vi "Pass State Machine.vi"   [LabVIEW 2013]
uses:
  typedefs/fg_typedef.ctl
  typedefs/subStates.ctl
  typedefs/DevRef Type.ctl
panel:
  # "A State Machine to Handle Passing"
types:
  T1 = typedef "subStates.ctl" = enum16{"null", "wait", "driver control", "auto", "manual override", "hold position", "rotate", "pickup", "pass", "load", "goto shoot", "shoot high goal", "shoot low goal", "cancel arm", "cancel shooter", "end"}
  T2 = typedef "fg_typedef.ctl" = enum16{"Get", "Set"}
  T3 = typedef "DevRef Type.ctl" = enum16{"Shooter Solenoid", "Latch Solenoid", "Right Up Sensor", "Right Down Sensor", "Hold Sensor", "2 Ball Switch", "Arm Encoder"}
  T4 = typedef "WPI_DigitalInputDevRef.ctl" = cluster{"DevStatus":errorcluster, "DIO Channel":T5, "Digital Module":T6}
  T5 = typedef "FPGA_DIOChannel.ctl" = enum8{"DIO 1", "DIO 2", "DIO 3", "DIO 4", "DIO 5", "DIO 6", "DIO 7", "DIO 8", "DIO 9", "DIO 10", "DIO 11", "DIO 12", "DIO 13", "DIO 14", "Invalid"}
  T6 = typedef "FPGA_TypedefDigitalModule.ctl" = enum16{"Digital Module 1", "Digital Module 2"}
  T7 = typedef "WPI_EncoderDevRef.ctl" = cluster{"DevStatus":errorcluster, "EncoderIndex":T8, "CounterIndex":T9, "DistancePerCount":dbl, "Decoding Type":T10}
  T8 = typedef "FPGA_EncoderIdx.ctl" = enum8{"Enc 0", "Enc 1", "Enc 2", "Enc 3", "Invalid"}
  T9 = typedef "FPGA_CounterCtrSystemIndex.ctl" = enum8{"Ctr 0", "Ctr 1", "Ctr 2", "Ctr 3", "Ctr 4", "Ctr 5", "Ctr 6", "Ctr 7", "Invalid"}
  T10 = typedef "WPI_EncoderType.ctl" = enum16{"1x", "2x", "4x"}
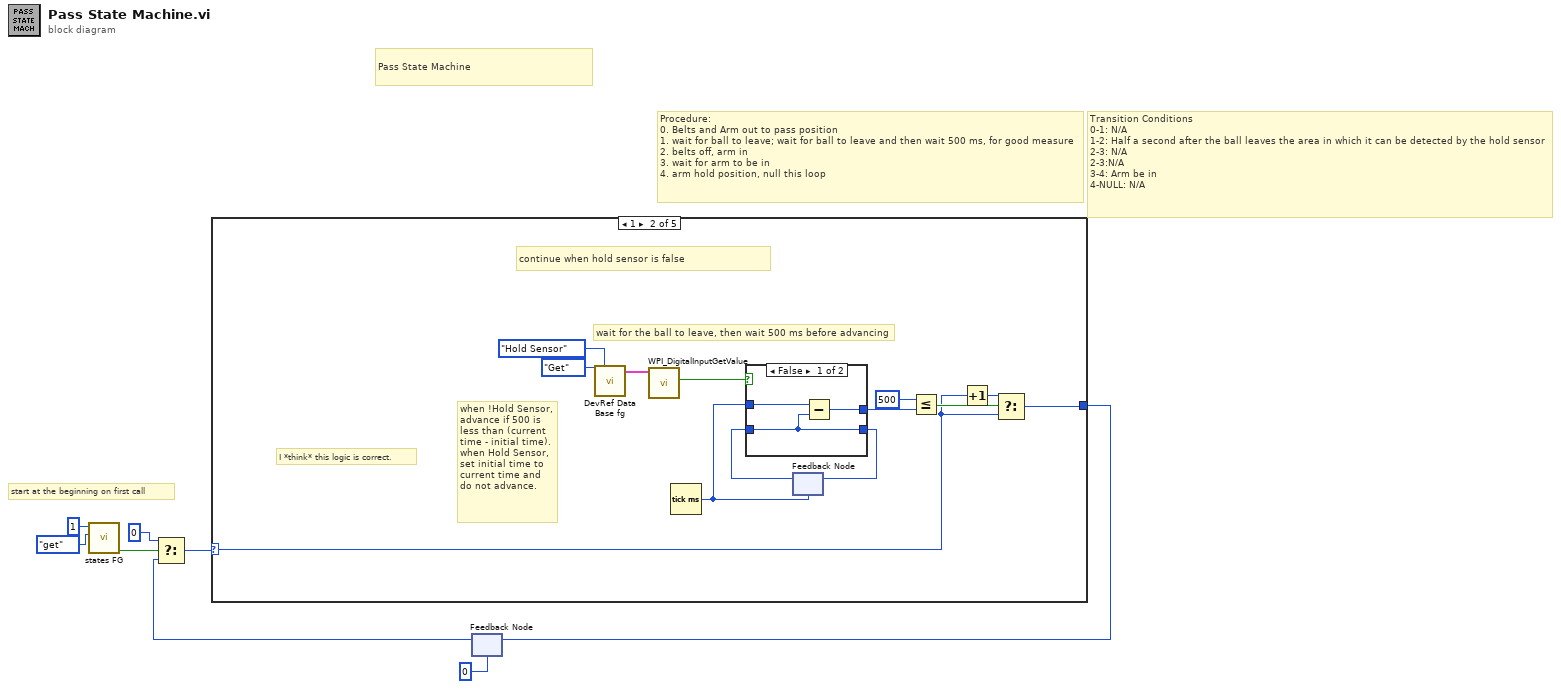
[diagram p0: block diagram]
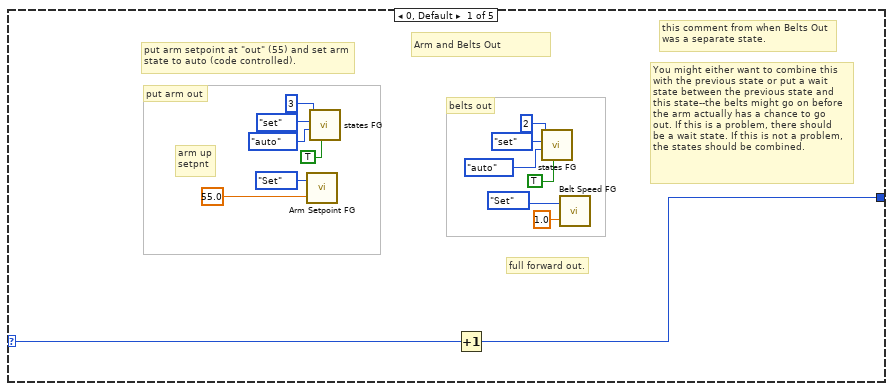
[diagram p2: hidden frame]
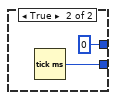
[diagram p3: hidden frame]
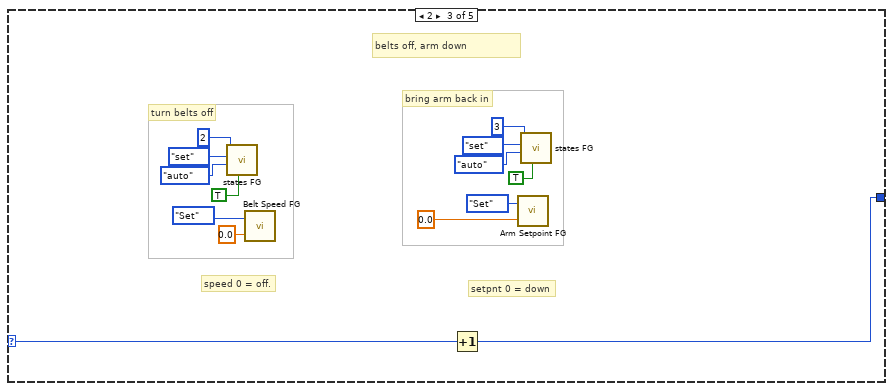
[diagram p4: hidden frame]
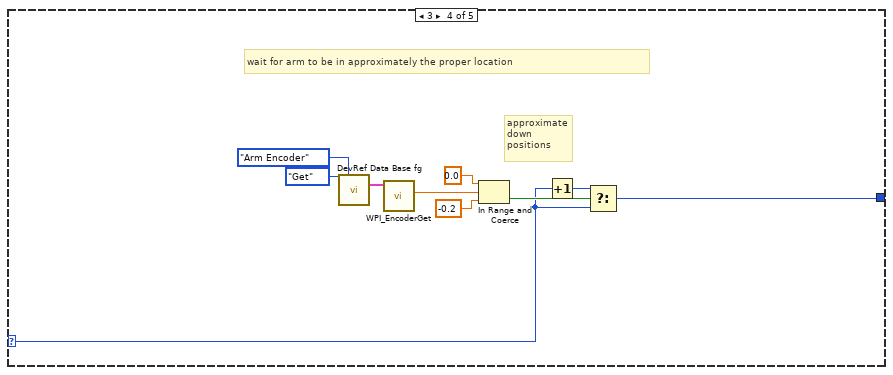
[diagram p5: hidden frame]
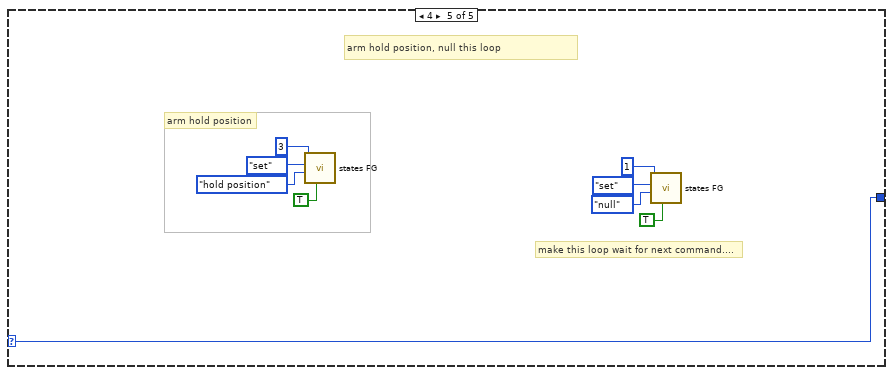
[diagram p6: hidden frame]
diagram:
  # "Transition Conditions\n0-1: N/A\n1-2: Half a second after the ball leaves the area in which it can be detected by the hold sensor\n2-3: N/A\n2-3:N/A\n3-4: Arm be in\n4-NULL: N/A"
  # "Procedure:\n0. Belts and Arm out to pass position\n1. wait for ball to leave; wait for ball to leave and then wait 500 ms, for good measure\n2. belts off, arm in\n3. wait for arm to be in\n4. arm hold position, null this loop"
  # "Pass State Machine"
  # "start at the beginning on first call"
  n1 = call "states FG.vi"("menu (get)"=enum16{"set", "get"}."get", "Loop ID"=1) -> ("first call?"=w1:bool)  [unwired: 6 in, 3 out]
  n2 = feedback #1(u8 0) -> (w4:u8)
  n3 = Select(t=u8 0, s=w1, f=w4) -> (s? t:f=w3:u8)
  n4 = case shown="1" w3 {
    selector: w3 -> [w17 w24 w44 w57 w65]
    tunnel: [w16 w23 w43 w55 w65] -> w7
    frame 0, Default {
      # "put arm out"
      # "full forward out."
      # "arm up\nsetpnt"
      # "this comment from when Belts Out\nwas a separate state."
      # "You might either want to combine this\nwith the previous state or put a wait\nstate between the previous state and\nthis state--the belts might go on before\nthe arm actually has a chance to go\nout. If this is a problem, there should\nbe a wait state. If this is not a problem,\nthe states should be combined."
      # "belts out"
      # "put arm setpoint at \"out\" (55) and set arm\nstate to auto (code controlled)."
      # "Arm and Belts Out"
      n5 = call "Arm Setpoint FG.vi"("Setpoint In"=55.0, "Menu"=fg_typedef."Set") -> ()  [unwired: 1 out]
      n6 = call "states FG.vi"("exit in"=TRUE, "subState in"=subStates."auto", "menu (get)"=enum16{"set", "get"}."set", "Loop ID"=3) -> ()  [unwired: 4 in, 4 out]
      n7 = Increment(x=w17) -> (x+1=w16:u8)
      n8 = call "states FG.vi"("exit in"=TRUE, "subState in"=subStates."auto", "menu (get)"=enum16{"set", "get"}."set", "Loop ID"=2) -> ()  [unwired: 4 in, 4 out]
      n9 = call "Belt Speed FG.vi"("Speed In"=1.0, "Menu"=fg_typedef."Set") -> ()  [unwired: 1 out]
    }
    frame 1 {
      # "continue when hold sensor is false"
      # "I *think* this logic is correct."
      # "when !Hold Sensor,\nadvance if 500 is\nless than (current\ntime - initial time).\nwhen Hold Sensor,\nset initial time to\ncurrent time and\ndo not advance."
      # "wait for the ball to leave, then wait 500 ms before advancing"
      n10 = call "DevRef Data Base fg.vi"("Menu"=fg_typedef."Get", "DevRef to Get"=DevRef_Type."Hold Sensor") -> ("Selected Sensor"=w26:T4)  [unwired: 23 in, 2 out]
      n11 = call <vilib>:"WPI_DigitalInputGetValue.vi"("DigitalInputDevRef"=w26) -> ("Value"=w28:bool)  [unwired: 8 in, 2 out]
      n12 = Tick Count (ms)() -> (millisecond timer value=w32:u32)
      n13 = feedback #2(w32) -> (w31:u32)
      n14 = case shown="False" w28 {
        tunnel: [w38 w40] -> w35
        tunnel: w31 -> [w38 _]
        tunnel: [w37 u32 0] -> w34
        tunnel: w32 -> [w36 _]
        frame False {
          n15 = Subtract(x=w36, y=w38) -> (x-y=w37:u32)
        }
        frame True {
          n16 = Tick Count (ms)() -> (millisecond timer value=w40:u32)
        }
      }
      n17 = feedback-in #2(w35) -> ()
      n18 = Less Or Equal?(x=u32 500, y=w34) -> (x <= y?=w30:bool)
      n19 = Increment(x=w24) -> (x+1=w29:u8)
      n20 = Select(t=w29, s=w30, f=w24) -> (s? t:f=w23:u8)
    }
    frame 2 {
      # "turn belts off"
      # "bring arm back in"
      # "setpnt 0 = down"
      # "speed 0 = off."
      # "belts off, arm down"
      n21 = call "states FG.vi"("exit in"=TRUE, "subState in"=subStates."auto", "menu (get)"=enum16{"set", "get"}."set", "Loop ID"=2) -> ()  [unwired: 4 in, 4 out]
      n22 = call "Belt Speed FG.vi"("Speed In"=0.0, "Menu"=fg_typedef."Set") -> ()  [unwired: 1 out]
      n23 = Increment(x=w44) -> (x+1=w43:u8)
      n24 = call "Arm Setpoint FG.vi"("Setpoint In"=0.0, "Menu"=fg_typedef."Set") -> ()  [unwired: 1 out]
      n25 = call "states FG.vi"("exit in"=TRUE, "subState in"=subStates."auto", "menu (get)"=enum16{"set", "get"}."set", "Loop ID"=3) -> ()  [unwired: 4 in, 4 out]
    }
    frame 3 {
      # "approximate\ndown\npositions"
      # "wait for arm to be in approximately the proper location"
      n26 = call "DevRef Data Base fg.vi"("Menu"=fg_typedef."Get", "DevRef to Get"=DevRef_Type."Arm Encoder") -> ("Selected Encoder"=w62:T7)  [unwired: 23 in, 2 out]
      n27 = call <vilib>:"WPI_EncoderGet.vi"("EncoderDevRef"=w62) -> ("Distance"=w61:dbl)  [unwired: 5 in, 5 out]
      n28 = In Range and Coerce(upper limit=0.0, x=w61, lower limit=-0.2) -> (In Range?=w58:bool)  [unwired: 1 out]
      n29 = Increment(x=w57) -> (x+1=w56:u8)
      n30 = Select(t=w56, s=w58, f=w57) -> (s? t:f=w55:u8)
    }
    frame 4 {
      # "arm hold position"
      # "make this loop wait for next command...."
      # "arm hold position, null this loop"
      n31 = call "states FG.vi"("exit in"=TRUE, "subState in"=subStates."hold position", "menu (get)"=enum16{"set", "get"}."set", "Loop ID"=3) -> ()  [unwired: 4 in, 4 out]
      n32 = call "states FG.vi"("exit in"=TRUE, "subState in"=subStates."null", "menu (get)"=enum16{"set", "get"}."set", "Loop ID"=1) -> ()  [unwired: 4 in, 4 out]
    }
  }
  n33 = feedback-in #1(w7) -> ()
